vi "Set Frequency.vi"(8 "error in (no error)":errorcluster, 9 "Synchronous":bool, 10 "Frequency":dbl format="%#_6pHz", 11 "Lock-in in":refnum<class "Lock-in.lvclass">) -> (0 "error out":errorcluster, 3 "Lock-in out":refnum<class "Lock-in.lvclass">)   [LabVIEW 2016, in "Lock-in.lvclass"]
uses:
  Lock-in.lvclass
  Lock-in.lvclass/Lock-in.ctl
  Read Lock-in driver.vi
  Write Lock-in driver.vi
  NHMFL_Core/Libraries/Instruments/Instrument Driver/Lock-in Driver/Lock-in Driver.lvclass
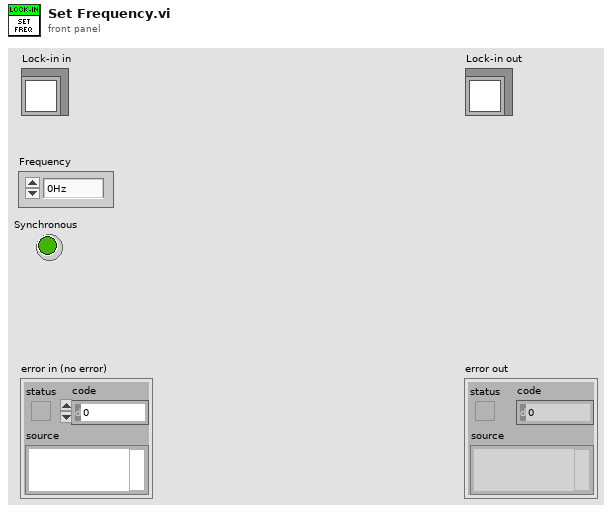
[diagram p1: front panel]
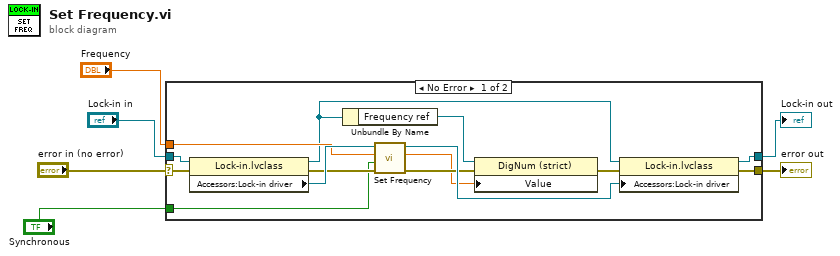
[diagram p0: block diagram]
diagram:
  n1 = case shown="No Error" "error in (no error)" {
    selector: "error in (no error)" -> [w19 w22]
    tunnel: [w13 w22] -> w5
    tunnel: [w14 w21] -> w3
    tunnel: "Lock-in in" -> [w20 w21]
    tunnel: "Frequency" -> [w17 _]
    tunnel: "Synchronous" -> [w7 _]
    frame No Error {
      n2 = property class="Lock-in.lvclass"(reference=w20, error in=w19) -> (reference out=w10:refnum<class "Lock-in.lvclass">, error out=w16:errorcluster, "Accessors:Lock-in driver"=w18:refnum<class "Lock-in Driver.lvclass">)
      n3 = Unbundle By Name(w10) -> ("Frequency ref"=w9:refnum<vi>)
      n4 = call-dynamic "Set Frequency.vi"("error in (no error)"=w16, "Synchronous"=w7, "Frequency"=w17, "Lock-in Driver in"=w18) -> ("error out"=w12:errorcluster, "Actual frequency"=w8:dbl, "Lock-in Driver out"=w15:refnum<class "Lock-in Driver.lvclass">)  [unwired: 5 in]
      n5 = property class="DigNum (strict)"(reference=w9, error in=w12, "Value"=w8) -> (error out=w11:errorcluster)  [unwired: 1 out]
      n6 = property class="Lock-in.lvclass"(reference=w10, error in=w11, "Accessors:Lock-in driver"=w15) -> (reference out=w14:refnum<class "Lock-in.lvclass">, error out=w13:errorcluster)
    }
    frame Error {
    }
  }
  "error out" <- w5
  "Lock-in out" <- w3
